vi "VF.vi"(4 "FieldLenght/2":dbl, 6 "GoalWidth/2":dbl, 7 "RobotY":dbl, 9 "BallY":dbl, 10 "BallX":dbl, 11 "RobotX":dbl) -> (3 "InsideCone":bool)   [LabVIEW 2018]
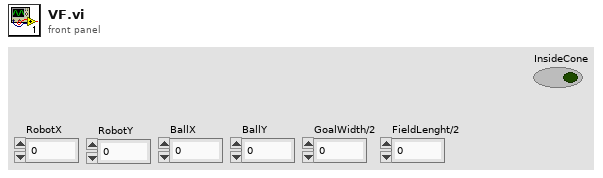
[diagram p1: front panel]
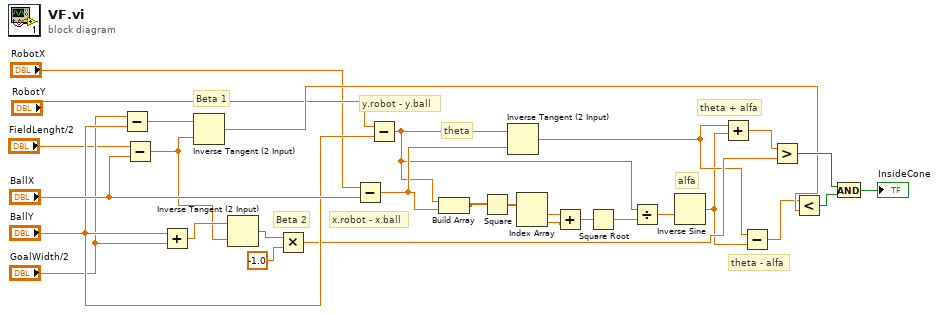
[diagram p0: block diagram]
diagram:
  # "theta - alfa"
  # "theta + alfa"
  # "theta"
  # "alfa"
  # "x.robot - x.ball"
  # "y.robot - y.ball"
  # "Beta 2"
  # "Beta 1"
  n1 = Subtract(x="GoalWidth/2", y="BallY") -> (x-y=w10:dbl)
  n2 = Subtract(x="FieldLenght/2", y="BallX") -> (x-y=w9:dbl)
  n3 = Add(x="BallY", y="GoalWidth/2") -> (x+y=w12:dbl)
  n4 = Inverse Tangent (2 Input)(1:w9, 2:w10) -> (0:w24:dbl)
  n5 = Inverse Tangent (2 Input)(1:w9, 2:w12) -> (0:w13:dbl)
  n6 = Multiply(x=w13, y=-1.0) -> (x*y=w22:dbl)
  n7 = Subtract(x="RobotX", y="BallX") -> (x-y=w2:dbl)
  n8 = Subtract(x="RobotY", y="BallY") -> (x-y=w1:dbl)
  n9 = Build Array(w1, w2) -> (w3:dbl[])
  n10 = Square(x=w3) -> (x^2=w8:dbl[])
  n11 = Inverse Tangent (2 Input)(1:w2, 2:w1) -> (0:w16:dbl)
  n12 = Index Array(array=w8) -> (element #1=w7:dbl, element #2=w6:dbl)  [unwired: 2 in]
  n13 = Add(x=w7, y=w6) -> (x+y=w5:dbl)
  n14 = Square Root(x=w5) -> (sqrt(x)=w4:dbl)
  n15 = Divide(x=w1, y=w4) -> (x/y=w17:dbl)
  n16 = Inverse Sine(1:w17) -> (0:w15:dbl)
  n17 = Add(x=w16, y=w15) -> (x+y=w21:dbl)
  n18 = Subtract(x=w16, y=w15) -> (x-y=w23:dbl)
  n19 = Greater?(x=w21, y=w22) -> (0:w26:bool)
  n20 = Less?(x=w23, y=w24) -> (x < y?=w25:bool)
  n21 = And(x=w26, y=w25) -> (x .and. y?=→"InsideCone":bool)
